vi "Configure Cool Output Limit.vi"(8 "error in (no error)":errorcluster, 10 "cool output limit, %":dbl=-100.0, 11 "HECR in":refnum<class "PL SMC HECR.lvclass">) -> (0 "error out":errorcluster, 3 "HECR out":refnum<class "PL SMC HECR.lvclass">)   [LabVIEW 2015, in "PL SMC HECR.lvclass"]
doc: "Configures cool output limit."
uses:
  PL SMC HECR.lvclass
  <vilib>/plasmapper/PL Modbus Client/PL Modbus Client.lvclass
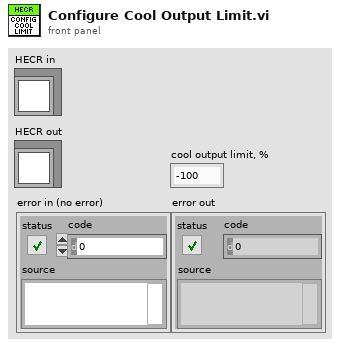
[diagram p1: front panel]
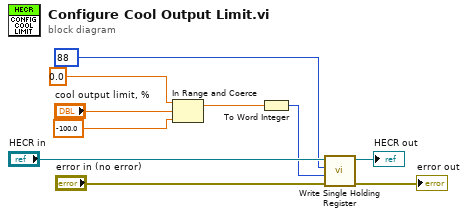
[diagram p0: block diagram]
diagram:
  n1 = In Range and Coerce(upper limit=0.0 ("Ttarget, °C"), x="cool output limit, %", lower limit=-100.0 ("Ttarget, °C")) -> (coerced(x)=w1:dbl)  [unwired: 1 out]
  n2 = To Word Integer(number=w1) -> (16bit integer=w2:i16)
  n3 = call <vilib>:"Write Single Holding Register.vi"("error in (no error)"="error in (no error)", "value"=w2, "address"=u16 88, "MODBUS in"="HECR in") -> ("error out"=→"error out":errorcluster, "MODBUS out"=→"HECR out":refnum<class "PL SMC HECR.lvclass">)  [unwired: 6 in]
